vi "GetNumberOfRecords.vi"(8 "error in (no error)":errorcluster, 11 "FpgaRefBase in":refnum<class "FpgaRefBase.lvclass">) -> (0 "error out":errorcluster, 2 "number of records":i32, 3 "FpgaRefBase out":refnum<class "FpgaRefBase.lvclass">)   [LabVIEW 2013, in "FpgaRefBase.lvclass"]
uses:
  FpgaRefBase.lvclass
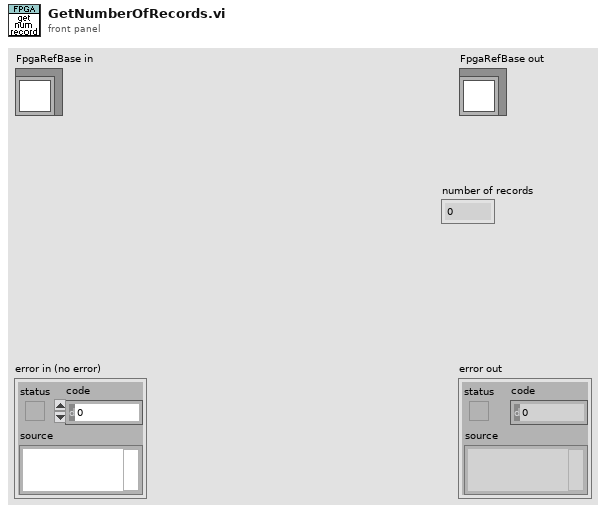
[diagram p1: front panel]
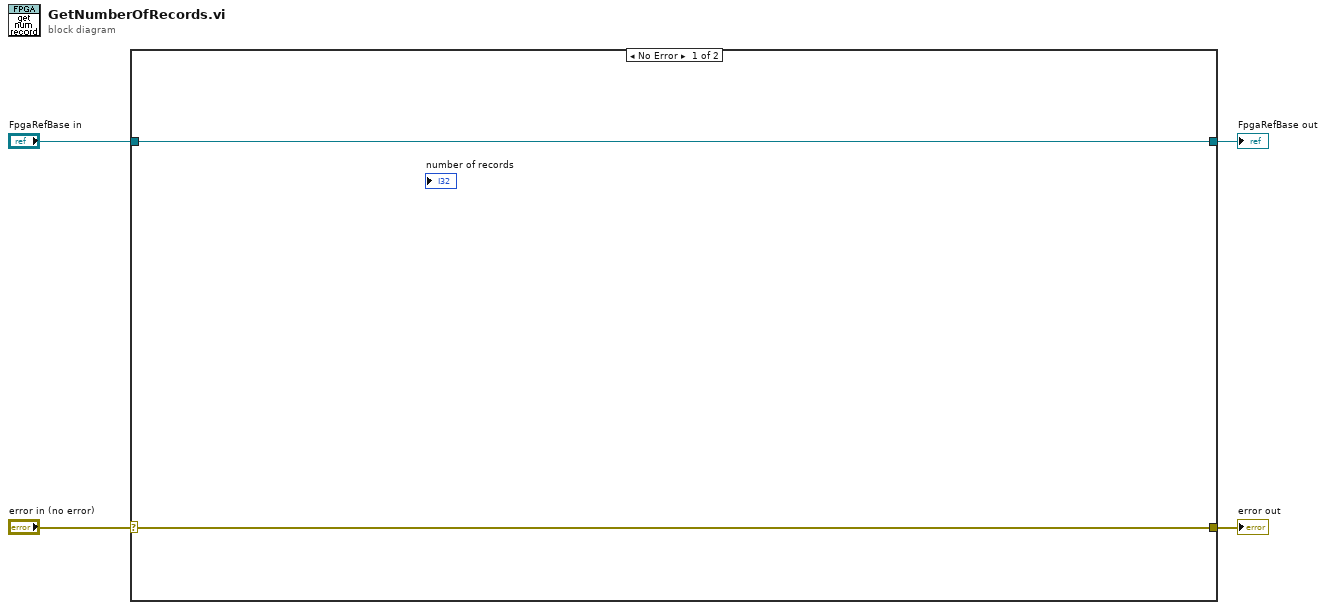
[diagram p0: block diagram]
diagram:
  n1 = case shown="No Error" "error in (no error)" {
    selector: "error in (no error)" -> [w5 w8]
    tunnel: [w5 w8] -> w3
    tunnel: [w6 w7] -> w1
    tunnel: "FpgaRefBase in" -> [w6 w7]
    frame No Error {
    }
    frame Error {
    }
  }
  "error out" <- w3
  "FpgaRefBase out" <- w1
